vi "SetCursorPos(x,y)NonLV.vi"(8 "error in":errorcluster, 11 "RelativePosition":cluster{"Horizontal":i32, "Vertical":i32}) -> (0 "error out":errorcluster, 3 "sucess":i32)   [LabVIEW 2013]
uses:
  user32.dll
  Linux VIs/guiLib.so
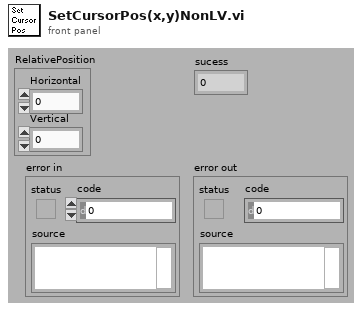
[diagram p1: front panel]
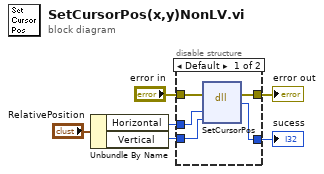
[diagram p0: block diagram]
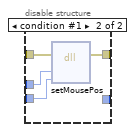
[diagram p2: hidden frame]
diagram:
  n1 = Unbundle By Name("RelativePosition") -> ("Horizontal"=w2:i32, "Vertical"=w3:i32)
  n2 = disable-structure shown="Default" {
    disable-tunnel: "error in" -> [w11 w15]
    disable-tunnel: [w10 w14] -> w5
    disable-tunnel: [w9 _] -> w4
    disable-tunnel: w3 -> [w8 w12]
    disable-tunnel: w2 -> [w7 w13]
    frame condition #0 (active) {
      n3 = dll-call lib="user32.*" fn="SetCursorPos"(error in=w11, "X"=w7, "Y"=w8) -> (error out=w10:errorcluster, "return type"=w9:i32)  [unwired: 4 in, 1 out]
    }
    frame condition #1 {
      n4 = dll-call lib="home/lvadmin/perforce/inmathed_lvcore-02_GUI/inmathed_lvcore-02_GUI/LabVIEWTestSystems/LV GUI ToolKit/LV GUI 2013/LabVIEW GUI Automation Toolkit/Utility/Linux VIs/guiLib.so" fn="setMousePos"(error in=w15, "x"=w13, "y"=w12) -> (error out=w14:errorcluster)  [unwired: 5 in, 1 out]
    }
  }
  "sucess" <- w4
  "error out" <- w5
